vi "NN_BBox_Get_Unique_Labels.vi"(7 "delimiter (\\t)":string="\t", 8 "error in (no error)":errorcluster, 11 "Anno File Paths":path[](array[path])) -> (0 "error out":errorcluster, 3 "Unique labels":string[](array[string]))   [LabVIEW 2020]
doc: "Returns unique labels from annotations in dataset."
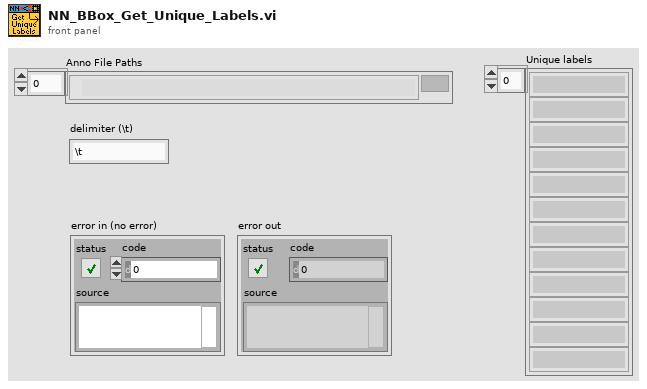
[diagram p1: front panel]
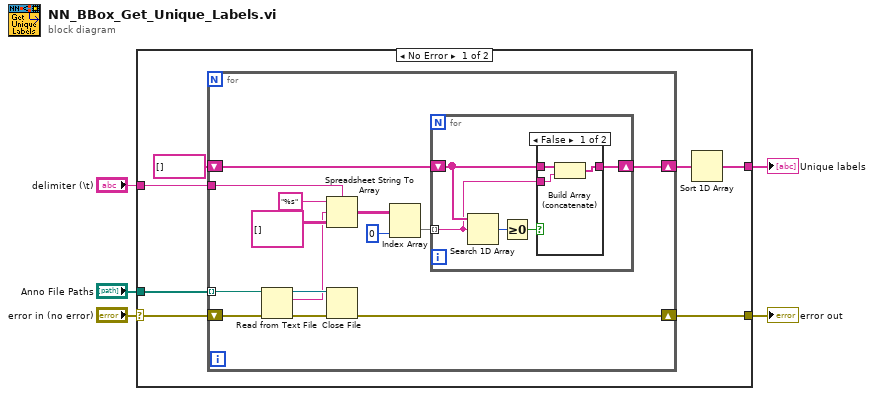
[diagram p0: block diagram]
diagram:
  n1 = case shown="No Error" "error in (no error)" {
    selector: "error in (no error)" -> [w9 w36]
    tunnel: [w6 _] -> w5
    tunnel: "delimiter (\\t)" -> [w10 _]
    tunnel: [w8 w36] -> w2
    tunnel: "Anno File Paths" -> [w7 _]
    frame No Error {
      n2 = for {
        shift-right: [w25] -> w12
        shift-left: string[] [] ("Classes[txt]") -> [w26]
        tunnel: w10 -> [w16]
        shift-right: [w14] -> w8
        shift-left: w9 -> [w15]
        tunnel: w7 -> [w13] mode=indexing
        n3 = Read from Text File(file (use dialog)=w13, error in=w15) -> (refnum out=w24:refnum<file>, text=w18:string, error out=w23:errorcluster)  [unwired: 2 in, 1 out]
        n4 = Spreadsheet String To Array(delimiter (Tab)=w16, format string="%s" ("format (%s)"), spreadsheet string=w18, array type (2D Dbl)=string[][] [] ("type (empty)")) -> (array=w22:string[][])
        n5 = Close File(refnum=w24, error in=w23) -> (error out=w14:errorcluster)  [unwired: 1 out]
        n6 = Index Array(array=w22, index (col)=0 ("disabled index (col)")) -> (element=w17:string[])  [unwired: 1 in]
        n7 = for {
          tunnel: w17 -> [w30] mode=indexing
          shift-right: [w28] -> w25
          shift-left: w26 -> [w31]
          n8 = Search 1D Array(1D array=w31, element=w30) -> (index of element=w29:i32)  [unwired: 1 in]
          n9 = Greater Or Equal To 0?(x=w29) -> (x >= 0?=w27:bool)
          n10 = case shown="False" w27 {
            tunnel: w30 -> [w32 _]
            tunnel: w31 -> [w34 w35]
            tunnel: [w33 w35] -> w28
            frame False {
              n11 = Build Array (concatenate)(w34, w32) -> (w33:string[])
            }
            frame True {
            }
          }
        }
      }
      n12 = Sort 1D Array(array=w12) -> (sorted array=w6:string[])
    }
    frame Error {
    }
  }
  "Unique labels" <- w5
  "error out" <- w2
